vi "chaveamento.vi"(0 "Pitot":dbl, 1 "hmin":dbl=15.0, 3 "hmax":dbl=20.0, 5 "Térmico":dbl, 11 "error in (no error)":errorcluster) -> (4 "chaveado":dbl, 6 "pitot":dbl, 8 "termico":dbl, 10 "Térmico?":bool, 15 "error out":errorcluster)   [LabVIEW 2017]
panel:
  in  "Tab Control":enum32{"Page 1", "Page 2"}(tab)
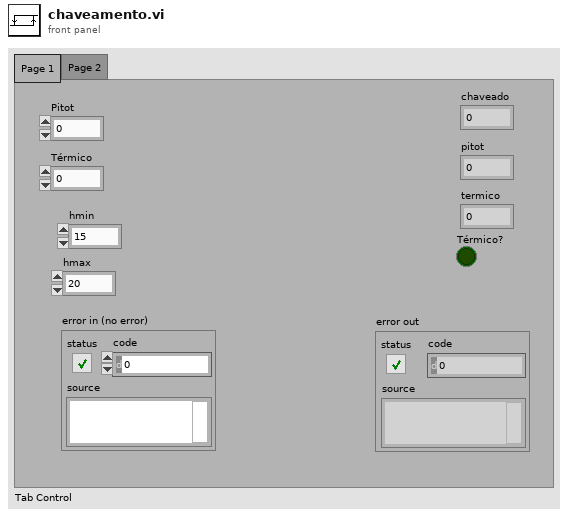
[diagram p1: front panel]
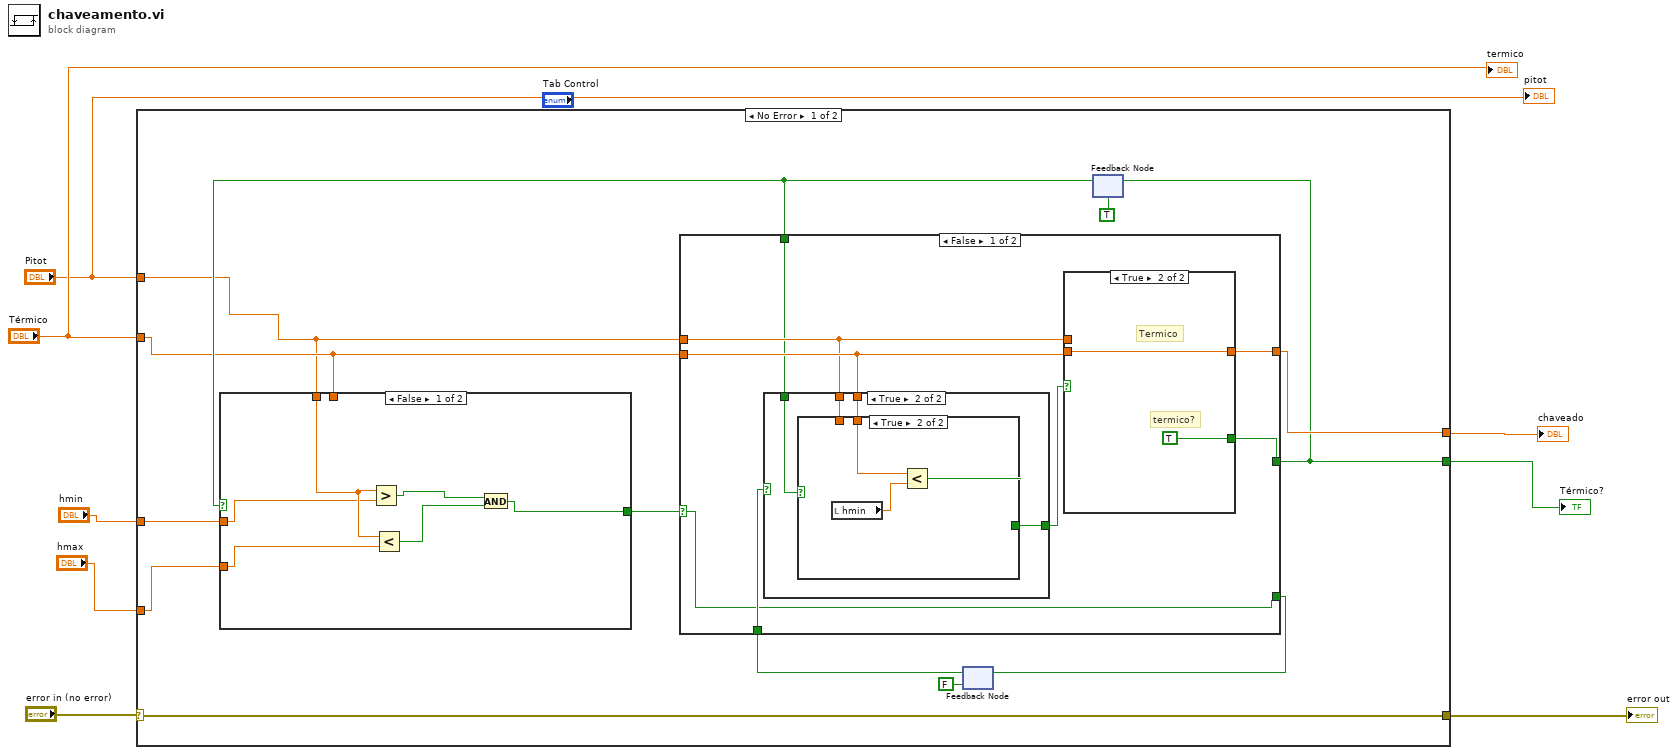
[diagram p0: block diagram]
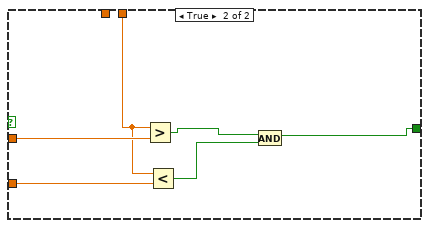
[diagram p2: hidden frame]
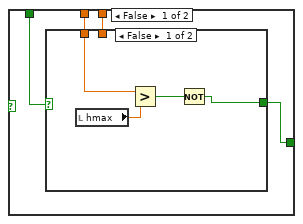
[diagram p3: hidden frame]
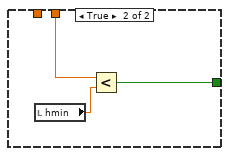
[diagram p4: hidden frame]
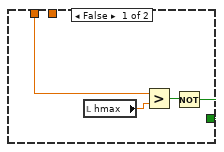
[diagram p5: hidden frame]
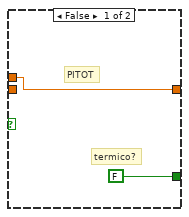
[diagram p6: hidden frame]
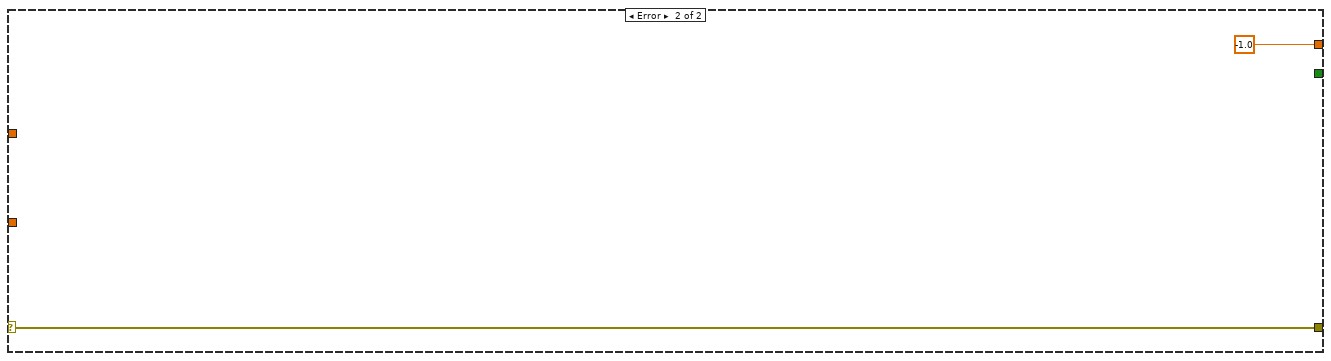
[diagram p9: hidden frame]
diagram:
  n1 = case shown="No Error" "error in (no error)" {
    selector: "error in (no error)" -> [w21 w78]
    tunnel: "Pitot" -> [w9 _]
    tunnel: "Térmico" -> [w13 _]
    tunnel: [w20 -1.0 ("y")] -> w4
    tunnel: [w21 w78] -> w7
    tunnel: "hmin" -> [w12 _]
    tunnel: "hmax" -> [w10 _]
    tunnel: [w18 _] -> w1
    frame No Error {
      n2 = feedback #1(FALSE) -> (w17:bool)
      n3 = feedback #2(TRUE) -> (w14:bool)
      n4 = case shown="False" w14 {
        tunnel: w13 -> [_ w32]
        tunnel: w12 -> [w24 w33]
        tunnel: [w22 w28] -> w11
        tunnel: w10 -> [w23 w31]
        tunnel: w9 -> [w25 _]
        frame False {
          n5 = Greater?(x=w25, y=w24) -> (0:w27:bool)
          n6 = Less?(x=w25, y=w23) -> (x < y?=w26:bool)
          n7 = And(x=w27, y=w26) -> (x .and. y?=w22:bool)
        }
        frame True {
          n8 = Greater?(x=w32, y=w33) -> (0:w30:bool)
          n9 = Less?(x=w32, y=w31) -> (x < y?=w29:bool)
          n10 = And(x=w30, y=w29) -> (x .and. y?=w28:bool)
        }
      }
      n11 = case shown="False" w11 {
        selector: w11 -> [w35 _]
        tunnel: w9 -> [w38 w72]
        tunnel: w13 -> [w39 w71]
        tunnel: [w41 w70] -> w20
        tunnel: [w40 w69] -> w18
        tunnel: w14 -> [w34 w68]
        tunnel: w17 -> [w36 _]
        tunnel: [w35 _] -> w16
        frame False {
          n12 = case shown="True" w36 {
            tunnel: w39 -> [w44 w56]
            tunnel: w38 -> [w42 w55]
            tunnel: [w43 w54] -> w37
            tunnel: w34 -> [w45 w53]
            frame False {
              n13 = case shown="False" w45 {
                tunnel: w44 -> [_ w52]
                tunnel: [w47 w50] -> w43
                tunnel: w42 -> [w46 _]
                frame False {
                  n14 = local read "hmax"() -> (w49:dbl)
                  n15 = Greater?(x=w46, y=w49) -> (0:w48:bool)
                  n16 = Not(x=w48) -> (.not. x?=w47:bool)
                }
                frame True {
                  n17 = local read "hmin"() -> (w51:dbl)
                  n18 = Less?(x=w52, y=w51) -> (x < y?=w50:bool)
                }
              }
            }
            frame True {
              n19 = case shown="True" w53 {
                tunnel: w56 -> [_ w63]
                tunnel: w55 -> [w60 _]
                tunnel: [w57 w61] -> w54
                frame False {
                  n20 = local read "hmax"() -> (w59:dbl)
                  n21 = Greater?(x=w60, y=w59) -> (0:w58:bool)
                  n22 = Not(x=w58) -> (.not. x?=w57:bool)
                }
                frame True {
                  n23 = local read "hmin"() -> (w62:dbl)
                  n24 = Less?(x=w63, y=w62) -> (x < y?=w61:bool)
                }
              }
            }
          }
          n25 = case shown="True" w37 {
            tunnel: w39 -> [_ w67]
            tunnel: [w65 w67] -> w41
            tunnel: w38 -> [w65 _]
            tunnel: [FALSE TRUE] -> w40
            frame False {
              # "termico?"
              # "PITOT"
            }
            frame True {
              # "termico?"
              # "Termico"
            }
          }
        }
        frame True {
          # "termico?"
          n26 = case shown="True" w68 {
            selector: w68 -> [w74 w75]
            tunnel: w72 -> [w73 _]
            tunnel: w71 -> [_ w76]
            tunnel: [w73 w76] -> w70
            tunnel: [w74 w75] -> w69
            frame False {
            }
            frame True {
            }
          }
        }
      }
      n27 = feedback-in #1(w16) -> ()
      n28 = feedback-in #2(w18) -> ()
    }
    frame Error {
    }
  }
  "chaveado" <- w4
  "error out" <- w7
  "Térmico?" <- w1
  "pitot" <- "Pitot"
  "termico" <- "Térmico"
